vi "evaluate.vi"(5 "Error shown?":bool, 7 "Node Path":string, 9 "Parse Tree In":T1) -> (1 "Was error?":bool, 2 "Result":string)   [LabVIEW 2021]
uses:
  <vilib>/National Instruments/Tree Map/Tree Map Data.ctl
  <vilib>/National Instruments/Tree Map/Tree Map.lvlib
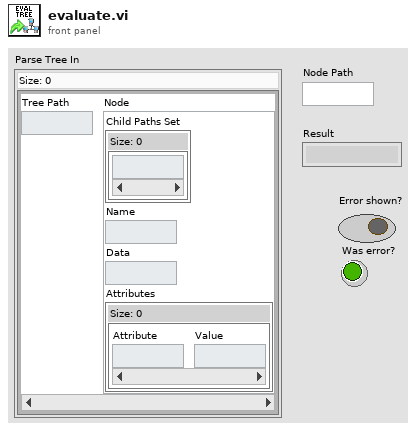
[diagram p1: front panel]
types:
  T1 = typedef "Tree Map.lvlib/Tree Map Data.ctl" = map{string, cluster{"Child Paths Set":set{string}, "Name":string, "Data":string, "Attributes":map{string, string}}}
  T2 = cluster{"Child Paths Set":set{string}, "Name":string, "Data":string, "Attributes":map{string, string}}
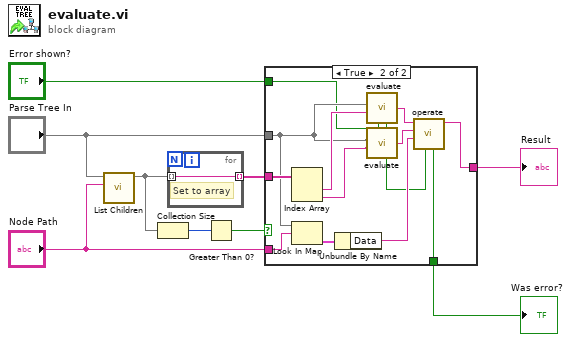
[diagram p0: block diagram]
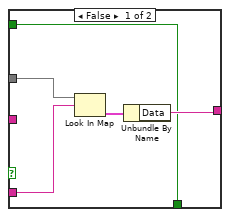
[diagram p2: hidden frame]
diagram:
  n1 = call <vilib>:"List Children.vi"("Tree Path"="Node Path", "Tree Map In"="Parse Tree In") -> ("Unique Child Paths Set"=w5:set{string})  [unwired: 9 in]
  n2 = Collection Size(1:w5) -> (0:w9:i32)
  n3 = for {
    tunnel: [w10] -> w4 mode=indexing
    tunnel: w5 -> [w10] mode=indexing
    # "Set to array"
  }
  n4 = Greater Than 0?(x=w9) -> (x > 0?=w8:bool)
  n5 = case shown="True" w8 {
    tunnel: "Parse Tree In" -> [w14 w20]
    tunnel: "Node Path" -> [w13 w27]
    tunnel: w4 -> [_ w29]
    tunnel: [w12 w26] -> w3
    tunnel: [w11 w24] -> w2
    tunnel: "Error shown?" -> [w11 w18]
    frame False {
      n6 = Look In Map(map=w14, key=w13) -> (value=w15:T2)  [unwired: 1 in, 1 out]
      n7 = Unbundle By Name(w15) -> ("Data"=w12:string)
    }
    frame True {
      n8 = Index Array(array=w29) -> (element #1=w23:string, element #2=w21:string)  [unwired: 2 in]
      n9 = Look In Map(map=w20, key=w27) -> (value=w28:T2)  [unwired: 1 in, 1 out]
      n10 = Unbundle By Name(w28) -> ("Data"=w25:string)
      n11 = call "evaluate.vi"("Error shown?"=w18, "Node Path"=w23, "Parse Tree In"=w20) -> ("Was error?"=w16:bool, "Result"=w22:string)  [unwired: 6 in]
      n12 = call "evaluate.vi"("Error shown?"=w16, "Node Path"=w21, "Parse Tree In"=w20) -> ("Was error?"=w17:bool, "Result"=w19:string)  [unwired: 6 in]
      n13 = call "operate.vi"("Error shown?"=w17, "a to b"=w25, "b"=w19, "a"=w22) -> ("Result"=w26:string, "Was error?"=w24:bool)  [unwired: 6 in]
    }
  }
  "Result" <- w3
  "Was error?" <- w2
